vi "Sigma_TriggerOut.vi"(7 "Axis(1)":i32=1, 8 "error in (no error)":errorcluster, 9 "Trigger distance (mm)":dbl=1.0, 10 "Travel per Pulse (mm)":dbl=0.004, 11 "VISA resource name":refnum<visa-resource-name>) -> (0 "error out":errorcluster, 3 "VISA resource name out":refnum<visa-resource-name>)   [LabVIEW 2018]
panel:
  out "resulting string":string
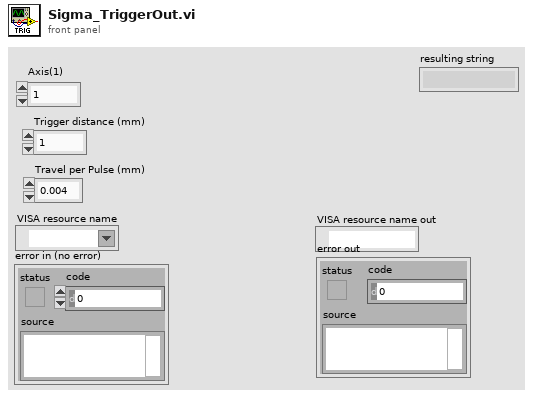
[diagram p1: front panel]
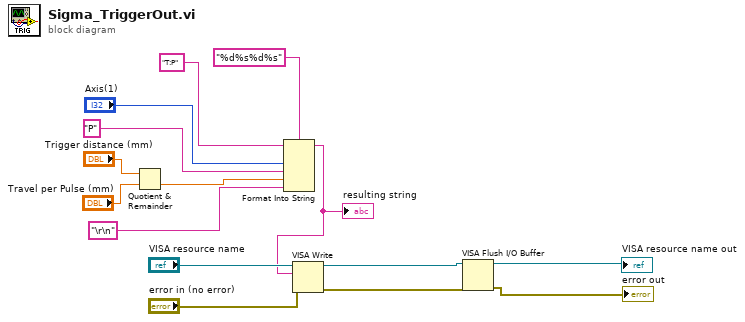
[diagram p0: block diagram]
diagram:
  n1 = Quotient & Remainder(x="Trigger distance (mm)", y="Travel per Pulse (mm)") -> (floor(x/y)=w6:dbl)  [unwired: 1 out]
  n2 = Format Into String(format string="%d%s%d%s", initial string="T:P", "Axis(1)", "P" ("input 2"), w6, "\r\n" ("input 3")) -> (resulting string=w12:string)  [unwired: 1 in, 1 out]
  "resulting string" <- w12
  n3 = VISA Write(VISA resource name="VISA resource name", write buffer=w12, error in (no error)="error in (no error)") -> (VISA resource name out=w5:refnum<visa-resource-name>, error out=w3:errorcluster)  [unwired: 1 out]
  n4 = VISA Flush I/O Buffer(VISA resource name=w5, error in (no error)=w3) -> (VISA resource name out=→"VISA resource name out":refnum<visa-resource-name>, error out=→"error out":errorcluster)  [unwired: 1 in]
